vi "run.vi"() -> ()   [LabVIEW 2012]
panel:
  out "w_R":dbl
  out "w_L":dbl
  out "MC_yi":dbl
  out "MC_xi":dbl
  out "distance":dbl
  out "MC_y":dbl
  out "MC_x":dbl
  out "V_My":dbl
  out "V_Mx":dbl
  in  "k":dbl
  in  "k_1":dbl
  in  "k_2":dbl
  out "MC":dbl
  out "gamma (deg)":dbl
  out "gamma (rad)":dbl
  out "MF":dbl
  in  "distance":dbl
  out "Beta (deg)":dbl
  out "cos_2alpha":dbl
  out "Shape Report (Shape Matching 1)[0].Centroid.x":sgl
  out "F_1B_1":dbl
  in  "stop":bool
  out "s":dbl
  out "Shape Report (Shape Matching 1)[0].Global Rectangle.x2Right":i32
  out "Shape Report (Shape Matching 1)[0].Global Rectangle.x1Left":i32
  out "A_1F":dbl
  out "A_1B_1":dbl
  out "F_1A_1":dbl
  out "Beta (rad)":dbl
  out "CF":dbl
  out "Image 2":T1(plugin-control)
  out "Image":T1(plugin-control)
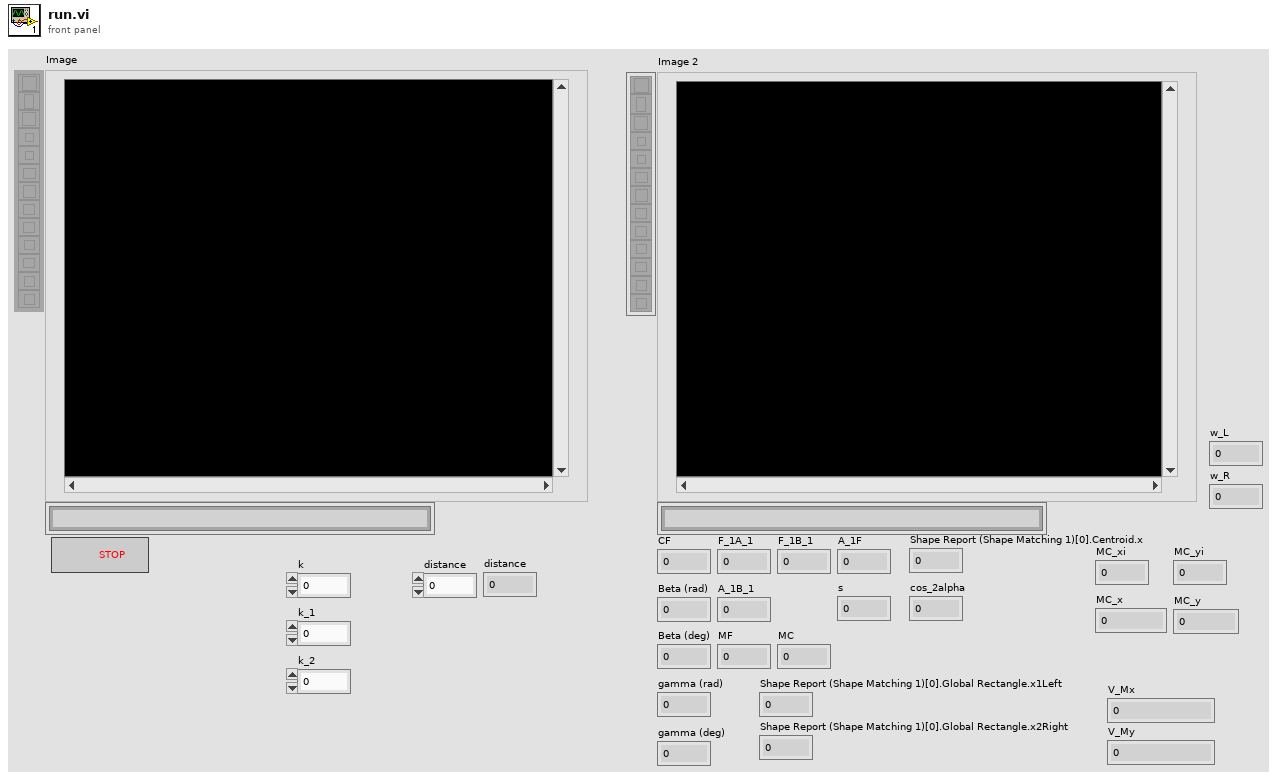
[diagram p1: front panel]
types:
  T1 = typedef "IMAQ Image.ctl" = refnum<image>
  T2 = cluster{"Global Rectangle":cluster{"x1Left":i32, "y1Top":i32, "x2Right":i32, "y2Bottom":i32}, "Centroid":cluster{"x":sgl, "y":sgl}, "Object Size":u32, "Score":dbl}[]
  T3 = cluster{"Shape Report (Shape Matching 1)[0]":cluster{"Global Rectangle":cluster{"x1Left":i32, "y1Top":i32, "x2Right":i32, "y2Bottom":i32}, "Centroid":cluster{"x":sgl, "y":sgl}, "Object Size":u32, "Score":dbl}, "Shape Report (Shape Matching 1)[1]":cluster{"Global Rectangle":cluster{"x1Left":i32, "y1Top":i32, "x2Right":i32, "y2Bottom":i32}, "Centroid":cluster{"x":sgl, "y":sgl}, "Object Size":u32, "Score":dbl}, "Shape Report (Shape Matching 1)[2]":cluster{"Global Rectangle":cluster{"x1Left":i32, "y1Top":i32, "x2Right":i32, "y2Bottom":i32}, "Centroid":cluster{"x":sgl, "y":sgl}, "Object Size":u32, "Score":dbl}, "Shape Report (Shape Matching 1)[3]":cluster{"Global Rectangle":cluster{"x1Left":i32, "y1Top":i32, "x2Right":i32, "y2Bottom":i32}, "Centroid":cluster{"x":sgl, "y":sgl}, "Object Size":u32, "Score":dbl}, "Shape Report (Shape Matching 1)[4]":cluster{"Global Rectangle":cluster{"x1Left":i32, "y1Top":i32, "x2Right":i32, "y2Bottom":i32}, "Centroid":cluster{"x":sgl, "y":sgl}, "Object Size":u32, "Score":dbl}, "Shape Report (Shape Matching 1)[5]":cluster{"Global Rectangle":cluster{"x1Left":i32, "y1Top":i32, "x2Right":i32, "y2Bottom":i32}, "Centroid":cluster{"x":sgl, "y":sgl}, "Object Size":u32, "Score":dbl}, "Shape Report (Shape Matching 1)[6]":cluster{"Global Rectangle":cluster{"x1Left":i32, "y1Top":i32, "x2Right":i32, "y2Bottom":i32}, "Centroid":cluster{"x":sgl, "y":sgl}, "Object Size":u32, "Score":dbl}, "Shape Report (Shape Matching 1)[7]":cluster{"Global Rectangle":cluster{"x1Left":i32, "y1Top":i32, "x2Right":i32, "y2Bottom":i32}, "Centroid":cluster{"x":sgl, "y":sgl}, "Object Size":u32, "Score":dbl}, "Shape Report (Shape Matching 1)[8]":cluster{"Global Rectangle":cluster{"x1Left":i32, "y1Top":i32, "x2Right":i32, "y2Bottom":i32}, "Centroid":cluster{"x":sgl, "y":sgl}, "Object Size":u32, "Score":dbl}}
  T4 = cluster{"x1Left":i32, "y1Top":i32, "x2Right":i32, "y2Bottom":i32}
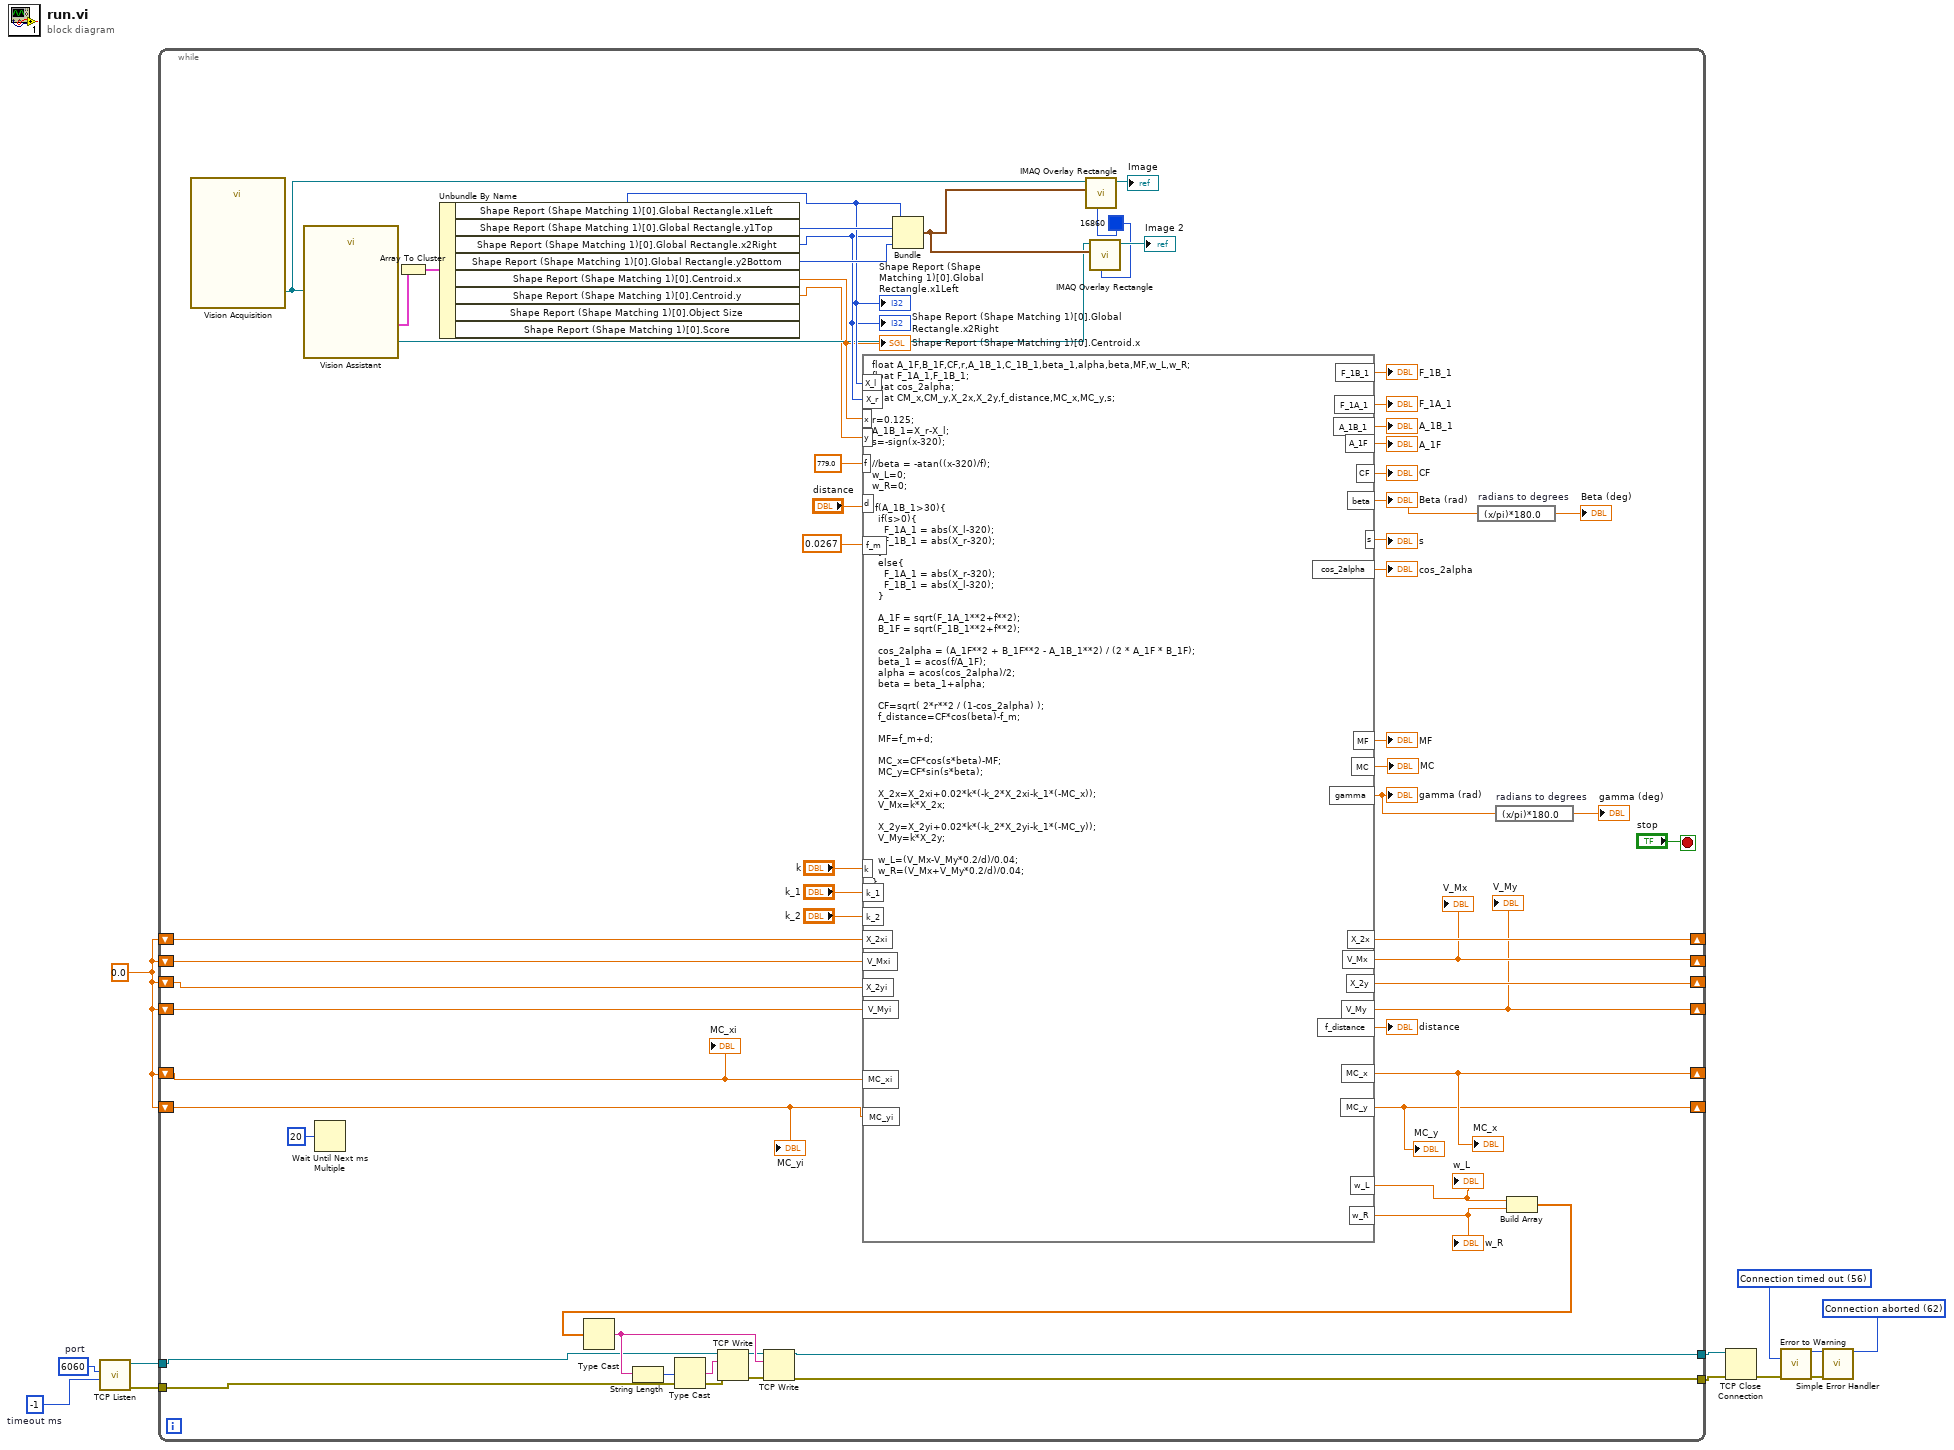
[diagram p0: block diagram]
diagram:
  w3 = 56 items=["No Error", "Argument Error", "Memory Full", "Out of Zone", "End of File", "File Already Open", "Generic File IO Error", "File Not Found", "File Permission Error", "Disk Full", "Duplicate Path", "Too Many Files Open", "Not Enabled", "Resource File Not Found", "Cannot Add Resource", "Resource Not Found", "Image Not Found", "Image Memory Error", "Pen Does Not Exist", "Config Bad Type", "Config Token Not Found", "Config Parse Error", "Config Memory Error", "Bad External Code Format", "Bad External Code Offset", "External Code Not Present", "Null Window", "Destroy Window Mixup", "Null Menu", "Print Aborted", "Bad Print Record", "Print Driver Error", "Windows Error During Print", "Memory Error During Print", "Print Dialog Error", "Generic Print Error", "Invalid Device Refnum", "Device Not Found", "Device Parameter Error", "Device Unit Error", "Can't Open Device", "Device Call Aborted", "Generic Error", "Cancelled By User", "Object ID Too Low", "Object ID Too High", "Object Not In Heap", "Unknown Heap", "Bad DefProc ID", "DefProc Not In Table", "Message Out Of Range", "Null Method", "Unknown Message", "Manager Call Not Supported", "Bad address", "Connection In progress", "Connection timed out", "Connection is already in progress", "Network attribute not supported", "Network error", "Address in use", "System out of memory", "Connection aborted", "Connection refused", "Connection is not connected", "Connection is already connected", "Connection closed", "Initialize error (interapplication manager)", "Bad occurrence", "Wait on unbound occurrence handler", "Occurrence queue overflow", "Bad path", "Semaphore not signaled", "Unrecognized type (interapplication manager)"] ("2nd Error to Convert")
  w4 = 62 items=["No Error", "Argument Error", "Memory Full", "Out of Zone", "End of File", "File Already Open", "Generic File IO Error", "File Not Found", "File Permission Error", "Disk Full", "Duplicate Path", "Too Many Files Open", "Not Enabled", "Resource File Not Found", "Cannot Add Resource", "Resource Not Found", "Image Not Found", "Image Memory Error", "Pen Does Not Exist", "Config Bad Type", "Config Token Not Found", "Config Parse Error", "Config Memory Error", "Bad External Code Format", "Bad External Code Offset", "External Code Not Present", "Null Window", "Destroy Window Mixup", "Null Menu", "Print Aborted", "Bad Print Record", "Print Driver Error", "Windows Error During Print", "Memory Error During Print", "Print Dialog Error", "Generic Print Error", "Invalid Device Refnum", "Device Not Found", "Device Parameter Error", "Device Unit Error", "Can't Open Device", "Device Call Aborted", "Generic Error", "Cancelled By User", "Object ID Too Low", "Object ID Too High", "Object Not In Heap", "Unknown Heap", "Bad DefProc ID", "DefProc Not In Table", "Message Out Of Range", "Null Method", "Unknown Message", "Manager Call Not Supported", "Bad address", "Connection In progress", "Connection timed out", "Connection is already in progress", "Network attribute not supported", "Network error", "Address in use", "System out of memory", "Connection aborted", "Connection refused", "Connection is not connected", "Connection is already connected", "Connection closed", "Initialize error (interapplication manager)", "Bad occurrence", "Wait on unbound occurrence handler", "Occurrence queue overflow", "Bad path", "Semaphore not signaled", "Unrecognized type (interapplication manager)"] ("1st Error to Convert")
  w9 = u16 6060  # port
  w10 = -1  # timeout ms
  w11 = 0.0 ("V_My")
  n1 = call <vilib>:"TCP Listen.vi"("timeout ms (wait forever: -1)"=w10, "port"=w9) -> ("error out"=w7:errorcluster, "connection ID"=w8:refnum<k5>)  [unwired: 5 in, 3 out]
  n2 = while {
    shift-right: [w41] -> _
    shift-left: w11 -> [w40]
    shift-right: [w42] -> _
    shift-left: w11 -> [w38]
    shift-right: [w43] -> _
    shift-left: w11 -> [w39]
    shift-right: [w44] -> _
    shift-left: w11 -> [w37]
    shift-right: [w30] -> _
    shift-left: w11 -> [w32]
    shift-right: [w29] -> _
    shift-left: w11 -> [w31]
    tunnel: w8 -> [w21]
    tunnel: w7 -> [w22]
    tunnel: [w20] -> w1
    tunnel: [w19] -> w2
    stop <- "stop" stop-if-true
    w45 = u32 16860 ("Color")
    n3 = call "Vision Acquisition"() -> ("Image Out"=w18:T1)  [unwired: 25 in, 2 out]
    n4 = call "Vision Assistant"("Image In"=w18) -> ("Image Out"=w16:T1, "Shape Report (Shape Matching 1)"=w17:T2)  [unwired: 23 in, 2 out]
    n5 = Wait Until Next ms Multiple(millisecond multiple=u32 20) -> ()  [unwired: 1 out]
    n6 = Array To Cluster(array=w17) -> (cluster=w71:T3)
    n7 = Unbundle By Name(w71) -> ("Shape Report (Shape Matching 1)[0].Global Rectangle.x1Left"=w67:i32, "Shape Report (Shape Matching 1)[0].Global Rectangle.y1Top"=w69:i32, "Shape Report (Shape Matching 1)[0].Global Rectangle.x2Right"=w66:i32, "Shape Report (Shape Matching 1)[0].Global Rectangle.y2Bottom"=w68:i32, "Shape Report (Shape Matching 1)[0].Centroid.x"=w65:sgl, "Shape Report (Shape Matching 1)[0].Centroid.y"=w15:sgl)  [unwired: 2 out]
    "Shape Report (Shape Matching 1)[0].Global Rectangle.x1Left" <- w67
    "Shape Report (Shape Matching 1)[0].Global Rectangle.x2Right" <- w66
    "Shape Report (Shape Matching 1)[0].Centroid.x" <- w65
    n8 = formula code="float A_1F,B_1F,CF,r,A_1B_1,C_1B_1,beta_1,alpha,beta,MF,w_L,w_R;\nfloat F_1A_1,F_1B_1;\nfloat cos_2alpha;\nfloat CM_x,CM_y,X_2x,X_2y,f_distance,MC_x,MC_y,s;\n\nr=0.125;\nA_1B_1=X_r-X_l;\ns=-sign(x-320);\n\n//beta = -atan((x-320)/f);\nw_L=0;\nw_R=0;\n\nif(A_1B_1>30){  \n  if(s>0){\n    F_1A_1 = abs(X_l-320);\n    F_1B_1 = abs(X_r-320);\n  }\n  else{\n    F_1A_1 = abs(X_r-320);\n    F_1B_1 = abs(X_l-320);\n  }\n\n  A_1F = sqrt(F_1A_1**2+f**2);\n  B_1F = sqrt(F_1B_1**2+f**2);\n \n  cos_2alpha = (A_1F**2 + B_1F**2 - A_1B_1**2) / (2 * A_1F * B_1F);\n  beta_1 = acos(f/A_1F);\n  alpha = acos(cos_2alpha)/2;\n  beta = beta_1+alpha;\n\n  CF=sqrt( 2*r**2 / (1-cos_2alpha) );\n  f_distance=CF*cos(beta)-f_m;\n\n  MF=f_m+d;\n\n  MC_x=CF*cos(s*beta)-MF;\n  MC_y=CF*sin(s*beta);\n\n  X_2x=X_2xi+0.02*k*(-k_2*X_2xi-k_1*(-MC_x));\n  V_Mx=k*X_2x;\n\n  X_2y=X_2yi+0.02*k*(-k_2*X_2yi-k_1*(-MC_y));\n  V_My=k*X_2y;\n\n  w_L=(V_Mx-V_My*0.2/d)/0.04;\n  w_R=(V_Mx+V_My*0.2/d)/0.04;\n}"("X_l"=w67, "X_r"=w66, "x"=w65, "y"=w15, "f"=779.0 ("input variable"), "d"="distance", "f_m"=0.0267 ("input variable"), "X_2yi"=w39, "X_2xi"=w37, "V_Mxi"=w38, "V_Myi"=w40, "k_2"="k_2", "k_1"="k_1", "k"="k", "MC_xi"=w32, "MC_yi"=w31) -> ("CF"=→"CF":dbl, "beta"=w56:dbl, "F_1A_1"=→"F_1A_1":dbl, "A_1B_1"=→"A_1B_1":dbl, "A_1F"=→"A_1F":dbl, "s"=→"s":dbl, "F_1B_1"=→"F_1B_1":dbl, "cos_2alpha"=→"cos_2alpha":dbl, "MF"=→"MF":dbl, "gamma"=w51:dbl, "MC"=→"MC":dbl, "X_2x"=w44:dbl, "X_2y"=w43:dbl, "V_Mx"=w42:dbl, "V_My"=w41:dbl, "f_distance"=→"distance":dbl, "MC_x"=w30:dbl, "MC_y"=w29:dbl, "w_L"=w13:dbl, "w_R"=w12:dbl)
    "Beta (rad)" <- w56
    "gamma (rad)" <- w51
    "V_Mx" <- w42
    "V_My" <- w41
    "MC_x" <- w30
    "MC_y" <- w29
    "w_L" <- w13
    "w_R" <- w12
    n9 = Bundle("x1Left"=w67, "y1Top"=w69, "x2Right"=w66, "y2Bottom"=w68) -> (w46:T4)  [unwired: 1 in]
    n10 = call "IMAQ Overlay Rectangle"("Color"=w45, "Rectangle"=w46, "Image"=w18) -> ("Image Out"=→"Image":T1)  [unwired: 7 in, 1 out]
    n11 = call "IMAQ Overlay Rectangle"("Color"=w45, "Rectangle"=w46, "Image"=w16) -> ("Image Out"=→"Image 2":T1)  [unwired: 7 in, 1 out]
    n12 = expression code="(x/pi)*180.0" "radians to degrees"(w56) -> (→"Beta (deg)":dbl)
    n13 = expression code="(x/pi)*180.0" "radians to degrees"(w51) -> (→"gamma (deg)":dbl)
    n14 = Build Array(w13, w12) -> (w14:dbl[])
    n15 = Type Cast(x=w14) -> (*(type *) &x=w27:string)  [unwired: 1 in]
    n16 = String Length(string=w27) -> (length=w25:i32)
    n17 = Type Cast(x=w25) -> (*(type *) &x=w26:string)  [unwired: 1 in]
    n18 = TCP Write(connection ID=w21, data in=w26, error in (no error)=w22) -> (connection ID out=w23:refnum<k5>, error out=w24:errorcluster)  [unwired: 1 in, 1 out]
    n19 = TCP Write(connection ID=w23, data in=w27, error in (no error)=w24) -> (connection ID out=w20:refnum<k5>, error out=w19:errorcluster)  [unwired: 1 in, 1 out]
    "MC_xi" <- w32
    "MC_yi" <- w31
  }
  n20 = TCP Close Connection(connection ID=w1, error in (no error)=w2) -> (error out=w6:errorcluster)  [unwired: 1 in, 1 out]
  n21 = call <vilib>:"Error to Warning.vi"("1st Error to Convert"=w4, "2nd Error to Convert"=w3, "error in"=w6) -> ("warning out"=w5:errorcluster)  [unwired: 12 in]
  n22 = call <vilib>:"Simple Error Handler.vi"("error in (no error)"=w5) -> ()  [unwired: 4 in, 5 out]
